vi "Shutdown.vi"(8 "error in":errorcluster, 11 "FPGA VI Reference Out":refnum<k20>) -> (0 "error out":errorcluster)   [LabVIEW 2017]
doc: "Shuts down the RT application."
uses:
  <vilib>/Utility/error.llb/Error Cluster From Error Code.vi
  <vilib>/rvi/errors/niLvFpgaAdjustHostInterfaceError.vi
  <vilib>/FPGAPlugInAG/Dynamic/niLvFpga_Close_Dynamic.vi
  <vilib>/rvi/interface/nirviReadWriteControl/nirviReadWriteControl.xnode
  <vilib>/rvi/interface/nirviCloseFPGA/nirviCloseFPGA.xnode
  <vilib>/NI_Real-Time Target Support.lvlib
  NiFpgaLv.dll
  <vilib>/rvi/interface/Simulation/niFpgaSimulationCallBeginRW.vi
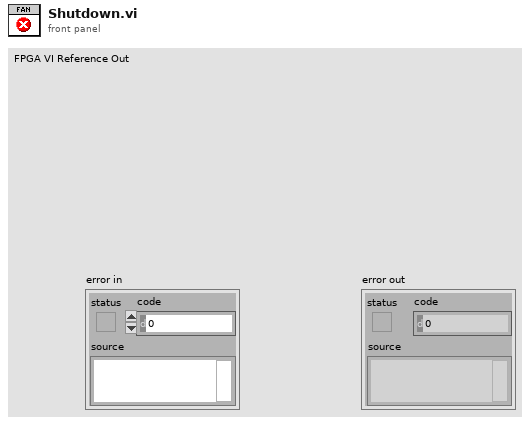
[diagram p1: front panel]
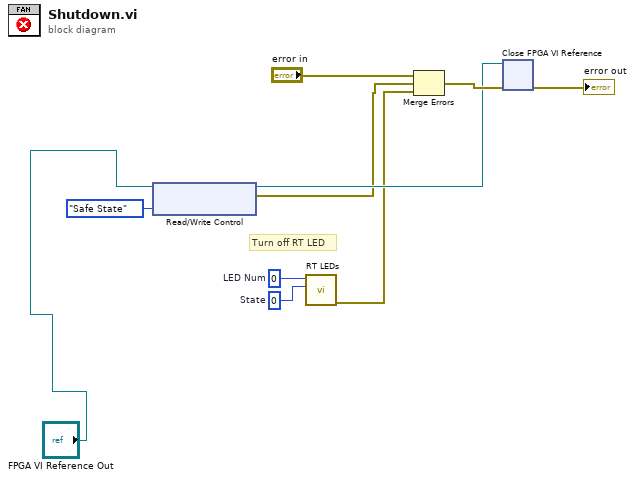
[diagram p0: block diagram]
diagram:
  w7 = 0  # State
  w8 = 0  # LED Num
  # "Turn off RT LED"
  n1 = xnode "Read/Write Control"("FPGA VI Reference In"="FPGA VI Reference Out", "New FPGA State"=enum16{"Safe State", "Control (PID)"}."Safe State" ("New FPGA state")) -> ("FPGA VI Reference Out"=w4:refnum<k20>, "error out"=w3:errorcluster)  [unwired: 1 in]
  n2 = call <vilib>:"RT LEDs.vi"("State"=w7, "LED Num"=w8) -> ("error out"=w2:errorcluster)  [unwired: 4 in, 1 out]
  n3 = Merge Errors("error in", w3, w2) -> (w9:errorcluster)
  n4 = xnode "Close FPGA VI Reference"("FPGA VI Reference In"=w4, "error in"=w9) -> ("error out"=→"error out":errorcluster)
